vi "ResonanceAnalyzer.vi"() -> ()   [LabVIEW 2015]
uses:
  <vilib>/imath/engines/lvmath2/RunTimeEngine/Managers/WorkSpace/UID Generator.vi
  <vilib>/imath/engines/lvmath2/RunTimeEngine/RangeToken/NIMS_Range_R2 - Float.vi
  <instcachedir>/0/NIMS_Range_R2 - Float_98052C3F8D284261A146188355820AF0.lvgen/NIMS_Range_R2 - Float_98052C3F8D284261A146188355820AF0_000.vi
  <vilib>/imath/engines/lvmath2/RunTimeEngine/CommandStatement/MC_CommandStatement_break.vi
  <vilib>/imath/engines/lvmath2/RunTimeEngine/RunTimeType/NIMS_RunTimeType_From StrictType (excl LVString).vi
  <instcachedir>/0/NIMS_RunTimeType_From StrictType (excl LVString)_EB1C38A9BC5048DA9ABDA8F781E54D21.lvgen/NIMS_RunTimeType_From StrictType (excl LVString)_EB1C38A9BC5048DA9ABDA8F781E54D21_000.vi
  <vilib>/imath/engines/lvmath2/RunTimeEngine/LocalVariableDefStatement/MC_LocalVariableDefStatement_Display.vi
  <vilib>/imath/engines/lvmath2/RunTimeEngine/RowToken/NIMS_RowToken_M_SorRV.vi
  <instcachedir>/0/NIMS_RowToken_M_SorRV_0ECFFCDE6465458AAAF8A8ED2D6C8AF1.lvgen/NIMS_RowToken_M_SorRV_0ECFFCDE6465458AAAF8A8ED2D6C8AF1_003.vi
  <vilib>/imathl/engines/lvmath/Functions/Error Handling/Create Error.vi
  <instcachedir>/0/NIMS_RowToken_M_SorRV_0ECFFCDE6465458AAAF8A8ED2D6C8AF1.lvgen/NIMS_RowToken_M_SorRV_0ECFFCDE6465458AAAF8A8ED2D6C8AF1_002.vi
  <vilib>/imath/engines/lvmath2/RunTimeEngine/BuiltInFunctions/randnormal/NIMS_randnormal(1,I32).vi
  <vilib>/imath/engines/lvmath2/RunTimeEngine/ErrorHandling/NIMS_Error From Error Code.vi
  <vilib>/imath/engines/lvmath2/RunTimeEngine/NodeEndStatement/NIMS_NodeEndStatement_Get Vector.vi
  <instcachedir>/0/NIMS_NodeEndStatement_Get Vector_ED7FC4F6B50246F79D573C75B2E51AF8.lvgen/NIMS_NodeEndStatement_Get Vector_ED7FC4F6B50246F79D573C75B2E51AF8_003.vi
  <vilib>/imath/engines/lvmath2/RunTimeEngine/VariableToken/NIMS_VariableToken_CondDefined.vi
  <instcachedir>/0/NIMS_VariableToken_CondDefined_FE30D0A1BFB24F098D41DEBABFE96BE1.lvgen/NIMS_VariableToken_CondDefined_FE30D0A1BFB24F098D41DEBABFE96BE1_003.vi
  <instcachedir>/0/NIMS_NodeEndStatement_Get Vector_ED7FC4F6B50246F79D573C75B2E51AF8.lvgen/NIMS_NodeEndStatement_Get Vector_ED7FC4F6B50246F79D573C75B2E51AF8_001.vi
  <vilib>/imath/engines/lvmath/Functions/Error Handling/MergeErrorsWrapper.vi
  <vilib>/imath/engines/lvmath2/RunTimeEngine/Managers/SymbolTable/Clear UID.vi
  <vilib>/imath/engines/lvmath2/RunTimeEngine/NodeEndStatement/NIMS_NodeEndStatement_Output.vi
  <instcachedir>/0/NIMS_NodeEndStatement_Output_53EC0D466D134D7ABD903AC30B43404B.lvgen/NIMS_NodeEndStatement_Output_53EC0D466D134D7ABD903AC30B43404B_005.vi
  <vilib>/imath/engines/lvmath2/RunTimeEngine/ErrorHandling/NIMS_Finalize Error.vi
  <vilib>/Utility/file.llb/Read Delimited Spreadsheet (DBL).vi
  <vilib>/imath/engines/lvmath2/RunTimeEngine/Managers/SymbolTable/NIMS_WorkSpace.lvlib
panel:
  out "Results":T1={"Amplitude"=1.0125354246286684, "Q"=10.011231515184043, "Center Freq"=599.8902895404412}
  out "XY Graph":cluster{"freq":dbl[], "Array":dbl[]}[](graph)=[{"freq"=[400.0, 401.0, 402.0, 403.0, 404.0, 405.0, 406.0, 407.0, 408.0, 409.0, 410.0, 411.0, 412.0, 413.0, 414.0, 415.0, 416.0, 417.0, 418.0, 419.0, 420.0, 421.0, 422.0, 423.0, 424.0, 425.0, 426.0, 427.0, 428.0, 429.0, 430.0, 431.0, 432.0, 433.0, 434.0, 435.0, 436.0, 437.0, 438.0, 439.0, 440.0, 441.0, 442.0, 443.0, 444.0, 445.0, 446.0, 447.0, 448.0, 449.0, 450.0, 451.0, 452.0, 453.0, 454.0, 455.0, 456.0, 457.0, 458.0, 459.0, 460.0, 461.0, 462.0, 463.0, 464.0, 465.0, 466.0, 467.0, 468.0, 469.0, 470.0, 471.0, 472.0, 473.0, 474.0, 475.0, 476.0, 477.0, 478.0, 479.0, 480.0, 481.0, 482.0, 483.0, 484.0, 485.0, 486.0, 487.0, 488.0, 489.0, 490.0, 491.0, 492.0, 493.0, 494.0, 495.0, 496.0, 497.0, 498.0, 499.0, 500.0, 501.0, 502.0, 503.0, 504.0, 505.0, 506.0, 507.0, 508.0, 509.0, 510.0, 511.0, 512.0, 513.0, 514.0, 515.0, 516.0, 517.0, 518.0, 519.0, 520.0, 521.0, 522.0, 523.0, 524.0, 525.0, 526.0, 527.0, 528.0, 529.0, 530.0, 531.0, 532.0, 533.0, 534.0, 535.0, 536.0, 537.0, 538.0, 539.0, 540.0, 541.0, 542.0, 543.0, 544.0, 545.0, 546.0, 547.0, 548.0, 549.0, 550.0, 551.0, 552.0, 553.0, 554.0, 555.0, 556.0, 557.0, 558.0, 559.0, 560.0, 561.0, 562.0, 563.0, 564.0, 565.0, 566.0, 567.0, 568.0, 569.0, 570.0, 571.0, 572.0, 573.0, 574.0, 575.0, 576.0, 577.0, 578.0, 579.0, 580.0, 581.0, 582.0, 583.0, 584.0, 585.0, 586.0, 587.0, 588.0, 589.0, 590.0, 591.0, 592.0, 593.0, 594.0, 595.0, 596.0, 597.0, 598.0, 599.0, 600.0, 601.0, 602.0, 603.0, 604.0, 605.0, 606.0, 607.0, 608.0, 609.0, 610.0, 611.0, 612.0, 613.0, 614.0, 615.0, 616.0, 617.0, 618.0, 619.0, 620.0, 621.0, 622.0, 623.0, 624.0, 625.0, 626.0, 627.0, 628.0, 629.0, 630.0, 631.0, 632.0, 633.0, 634.0, 635.0, 636.0, 637.0, 638.0, 639.0, 640.0, 641.0, 642.0, 643.0, 644.0, 645.0, 646.0, 647.0, 648.0, 649.0, 650.0, 651.0, 652.0, 653.0, 654.0, 655.0, 656.0, 657.0, 658.0, 659.0, 660.0, 661.0, 662.0, 663.0, 664.0, 665.0, 666.0, 667.0, 668.0, 669.0, 670.0, 671.0, 672.0, 673.0, 674.0, 675.0, 676.0, 677.0, 678.0, 679.0, 680.0, 681.0, 682.0, 683.0, 684.0, 685.0, 686.0, 687.0, 688.0, 689.0, 690.0, 691.0, 692.0, 693.0, 694.0, 695.0, 696.0, 697.0, 698.0, 699.0, 700.0, 701.0, 702.0, 703.0, 704.0, 705.0, 706.0, 707.0, 708.0, 709.0, 710.0, 711.0, 712.0, 713.0, 714.0, 715.0, 716.0, 717.0, 718.0, 719.0, 720.0, 721.0, 722.0, 723.0, 724.0, 725.0, 726.0, 727.0, 728.0, 729.0, 730.0, 731.0, 732.0, 733.0, 734.0, 735.0, 736.0, 737.0, 738.0, 739.0, 740.0, 741.0, 742.0, 743.0, 744.0, 745.0, 746.0, 747.0, 748.0, 749.0, 750.0, 751.0, 752.0, 753.0, 754.0, 755.0, 756.0, 757.0, 758.0, 759.0, 760.0, 761.0, 762.0, 763.0, 764.0, 765.0, 766.0, 767.0, 768.0, 769.0, 770.0, 771.0, 772.0, 773.0, 774.0, 775.0, 776.0, 777.0, 778.0, 779.0, 780.0, 781.0, 782.0, 783.0, 784.0, 785.0, 786.0, 787.0, 788.0, 789.0, 790.0, 791.0, 792.0, 793.0, 794.0, 795.0, 796.0, 797.0, 798.0, 799.0, 800.0], "Array"=[0.10740244651787122, 0.15281838289829783, 0.08959115748735166, 0.14809526149818455, 0.13102686084532728, 0.1104993829827506, 0.1221783389006147, 0.15050889317348842, 0.12029736326487445, 0.13037718741363646, 0.15243658974820584, 0.1374153902648614, 0.10978943923875586, 0.11543254265874583, 0.116749384195053, 0.15255299393630767, 0.12857585311403671, 0.11097529559717934, 0.1350388671955145, 0.14129997658045362, 0.16703549012694668, 0.14056905939318204, 0.15670938293701409, 0.1745965004264096, 0.15263763075519182, 0.1538378456426476, 0.1655560882427844, 0.15042578416569982, 0.17077928893541036, 0.14546868063086157, 0.1284127118932754, 0.14499346079719164, 0.14922747914991136, 0.1776417666138386, 0.14486375149154065, 0.1514964505869006, 0.1423909822834546, 0.1221032080951852, 0.12573244654842436, 0.16394597483895484, 0.18819152291011748, 0.15653899730011506, 0.12231585004152735, 0.13837823070137883, 0.1820668469920245, 0.16117180400928585, 0.18404838769308257, 0.18388021368066343, 0.148855772839171, 0.16783333316882265, 0.15503774605936327, 0.16367980030790852, 0.1579857648450566, 0.18191502199890683, 0.18970595823297254, 0.1944117552163931, 0.17266173161962406, 0.1802135947011225, 0.17855434351423938, 0.20062811939961647, 0.20654642108343524, 0.2052027035839432, 0.14902958539641598, 0.1762033423674224, 0.18327011348703162, 0.2283954425279633, 0.21827276447564503, 0.17754461590565587, 0.1892535385196978, 0.17952124670585873, 0.20008031880994345, 0.18189891897781724, 0.19794893957248644, 0.17613003418044218, 0.2249405249742432, 0.2121694451348723, 0.236670289359744, 0.2122005230430719, 0.1991946566567743, 0.212989347219985, 0.1787092964007292, 0.23389290334086227, 0.21930355311221128, 0.2559430561689233, 0.2107510422017375, 0.2213373501904825, 0.23459650705845927, 0.23411604572589576, 0.24232120185154685, 0.2579793486248234, 0.2558574257254317, 0.20496503693873555, 0.23239561943384532, 0.20896666579796563, 0.2614634805616313, 0.2258417261954543, 0.2471379676293738, 0.29307296878981853, 0.26178804891270624, 0.28960879040736437, 0.2788051456775778, 0.2737419120741029, 0.2784378688053793, 0.27898009359666054, 0.2915181736906019, 0.3033190946663929, 0.3000947700143919, 0.29665578583792496, 0.27482781058991157, 0.276171909679604, 0.27867649313953385, 0.2900655139885531, 0.2847266539584309, 0.2827978296624287, 0.31246587606549975, 0.3182942076336981, 0.2996410250956576, 0.32466743458622577, 0.3200048633179981, 0.31396337632360016, 0.3383915715497288, 0.32037493481420787, 0.34373662643485814, 0.3766872010424195, 0.34832133013105215, 0.33889616380084375, 0.4074268521903415, 0.34953183194534726, 0.33611613987777045, 0.39974131071551966, 0.3566730066279571, 0.34703115551990643, 0.3968775547607246, 0.4043501402167882, 0.3761696888376735, 0.3948411944517424, 0.3690359877672123, 0.43399509946970144, 0.43673286069535106, 0.39641181561210903, 0.4137969831790379, 0.4617765348706966, 0.4726295604520662, 0.4261537242721796, 0.4514042366383567, 0.45426474364682407, 0.45154083243783616, 0.49668249205938647, 0.4672454873406263, 0.5048940014747391, 0.5130668244433702, 0.5416562561443161, 0.5268395198682813, 0.5320264594999139, 0.546074355673345, 0.5251244571563372, 0.5744842802378644, 0.581350604617343, 0.5795838749124972, 0.5623338651916296, 0.5935843524297746, 0.5894221188352807, 0.6062038075829269, 0.6417195251539344, 0.634690715231069, 0.651868808006857, 0.6677428951850922, 0.6633513933529221, 0.6926614547702747, 0.6789450971670071, 0.7004064565103679, 0.6988271486328266, 0.7249285790621133, 0.7576714767505519, 0.7933063177685261, 0.8042720699856534, 0.7740231288836648, 0.7908060031158608, 0.8348634973967137, 0.844537787339374, 0.8400940710471335, 0.8482714179186746, 0.8432113148306352, 0.8703815460446738, 0.8968823832449301, 0.8715528206370958, 0.9308369472650522, 0.946983134130226, 0.9331356861843558, 0.9310495156756244, 0.9578146226109034, 0.9899983028755162, 0.9934759739042415, 0.9865124430027351, 1.0198994221003552, 0.9793454680620476, 1.040723912454541, 1.0019829426536175, 0.9878851948437057, 0.9931436118790047, 0.9998997955421117, 1.0241340949804192, 0.9980604879191322, 1.0004059988811909, 0.9964311453849393, 1.035115606150817, 1.014821095046213, 0.9889263917806297, 1.0179292524113845, 0.9605549119859166, 0.9560504690148568, 0.922530600901802, 0.9022757533720215, 0.9183222779288016, 0.9048488262003115, 0.9071789367812199, 0.9289015802343044, 0.8485576784792067, 0.8417815720374748, 0.8631395677579252, 0.8802707620426905, 0.8239894591940262, 0.8194511336977124, 0.7907852548996013, 0.813393533100567, 0.7813841594826026, 0.7335140123481045, 0.7690250917543924, 0.7661270744942449, 0.7081428294002305, 0.7275011248548809, 0.7288470799197462, 0.7310329276991778, 0.6858348894016951, 0.6545573028680088, 0.6640132244545103, 0.644157127864353, 0.6291484828008138, 0.6394589009817717, 0.6067453989698446, 0.6532855868688, 0.6161204004806324, 0.6150443381543468, 0.604273501743808, 0.6142461968037111, 0.5478912448786132, 0.5436770383181866, 0.5595910875659509, 0.5663136233109691, 0.5726300741195651, 0.5374425496882539, 0.5331011268367872, 0.49814276248296235, 0.5168627643519728, 0.49766324611051416, 0.494509126918839, 0.44464226610264207, 0.46929064541696053, 0.5205436518966415, 0.47456930528748426, 0.4273781407761661, 0.500119758518092, 0.5073860051476381, 0.4522174778467483, 0.43540532391181086, 0.4277470264905283, 0.45017848944633887, 0.38725813822260935, 0.43674588843293044, 0.42458002025502534, 0.4127836504534946, 0.4103666012150693, 0.40156767957870654, 0.39257867428810883, 0.40667705195073284, 0.43063546042850814, 0.3659919078706112, 0.40972523395198057, 0.40736834646343606, 0.4007217107777696, 0.3775120158678112, 0.35347247408739463, 0.3665994653344173, 0.35075199676799695, 0.32756109923258453, 0.37819715452738345, 0.35086941336678446, 0.35364004526844284, 0.3508398401104885, 0.3278260030576613, 0.32606974975065, 0.36441220206503216, 0.3440542864177623, 0.33103347985615655, 0.34576209714919515, 0.29092039816816706, 0.322274373671659, 0.3289061621350945, 0.30706296086408164, 0.3356218820756341, 0.32657661683896744, 0.2718225279989093, 0.32117955239798424, 0.30421160254751883, 0.27488395739312743, 0.2699908334822933, 0.2974915668952296, 0.28030899970393053, 0.27808804851581603, 0.24958907402046104, 0.27752879200285546, 0.28798032098818105, 0.2899865558922329, 0.254155342047928, 0.27433746535894193, 0.2966394614788142, 0.2650608715264895, 0.25932977780652283, 0.26487880078924225, 0.28141762463064746, 0.24233375708797547, 0.26702591219274524, 0.27655649784368713, 0.2749902813664165, 0.30379696818985197, 0.23350986845042287, 0.2914434978036537, 0.2548922376708591, 0.23154428185303677, 0.2693647169174003, 0.246150843221038, 0.24582181840925713, 0.2683660789256584, 0.25505675230040076, 0.25502826942985396, 0.27409213618113265, 0.22923011909348115, 0.23902506489589356, 0.2263346242039908, 0.21302480728051618, 0.23727434998850835, 0.2262192765545401, 0.21310004964379087, 0.248655475562663, 0.20180136113191977, 0.2122401027267436, 0.2509455407040858, 0.230264588483497, 0.20250360523920458, 0.22731653665623414, 0.2490361788808062, 0.22643826343509388, 0.22968142184378812, 0.228650289735457, 0.17747612924159473, 0.19587939404704874, 0.2365709003275931, 0.2207676659030181, 0.22120487822560841, 0.18393665061567777, 0.21599364522205494, 0.19373202283935284, 0.23389465084970545, 0.22983528539400916, 0.19334916599901192, 0.19245765890172797, 0.22578301105299753, 0.19775413579077106, 0.17816726939045804, 0.18966882935080356, 0.18760245648961316, 0.1914780125451503, 0.23305415087844095, 0.2143436771140928, 0.18712407047353985, 0.18032134679831235, 0.19347382576694527, 0.21362119150828224, 0.20185364505963843, 0.20433145754719834, 0.20329667400716067, 0.19029914718681923, 0.1591216111307436, 0.19208811147022664, 0.1926714623146115, 0.1597415120392497, 0.1852098930696274, 0.18637084164384937, 0.19146388692811167, 0.20547364695786818, 0.17863226190779827, 0.15695795749571714, 0.18214109732385403, 0.17367128443407268, 0.1613401334142838, 0.1700049889142177, 0.17999562799846414, 0.18759946320178397, 0.19154195290156165, 0.17609562635859496, 0.16345341866704946]}, ...(2 in all)]
  in  "Tab Control":enum32{"Simulated", "Experiment"}(tab)
  in  "df":dbl=0.314159
  in  "Q":dbl=10.0
  in  "Center Freq":dbl=600.0
  in  "Start Freq":dbl=400.0
  in  "End Freq":dbl=800.0
  in  "Noise Level":dbl=0.02
  in  "Filename":path
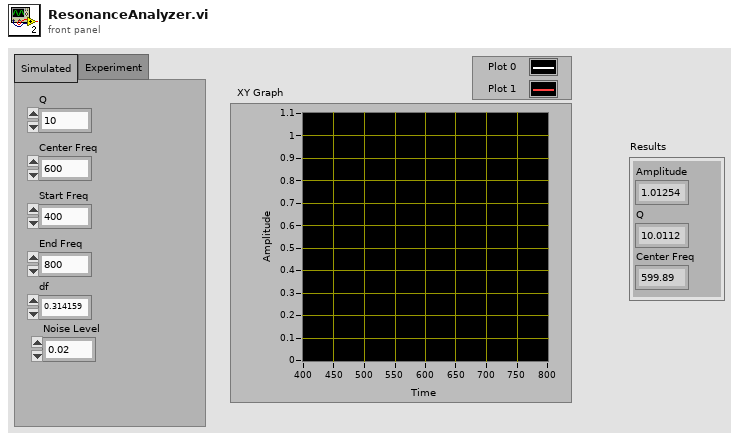
[diagram p1: front panel]
types:
  T1 = cluster{"Amplitude":dbl, "Q":dbl, "Center Freq":dbl}
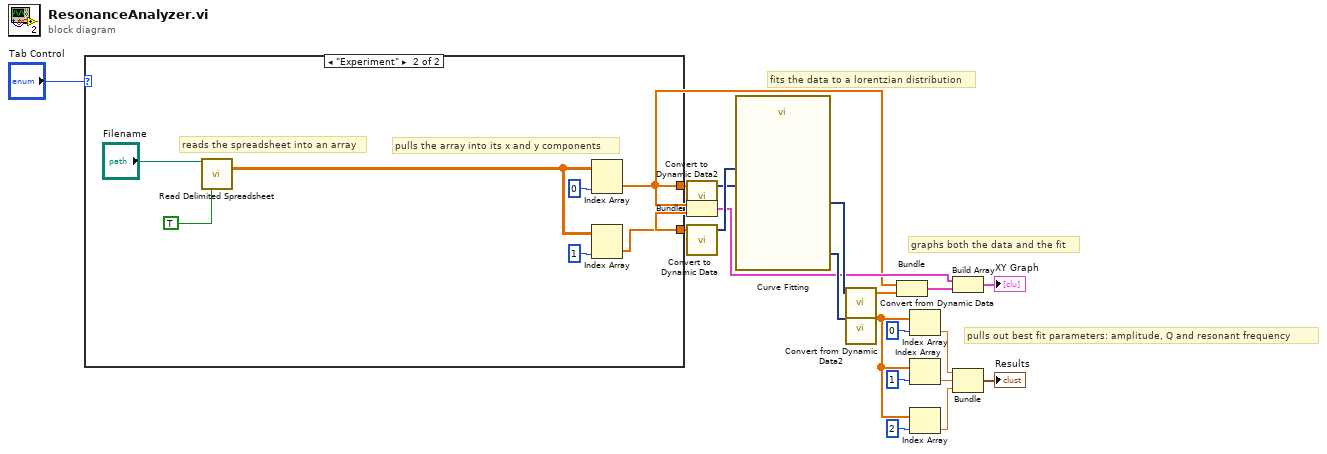
[diagram p0: block diagram]
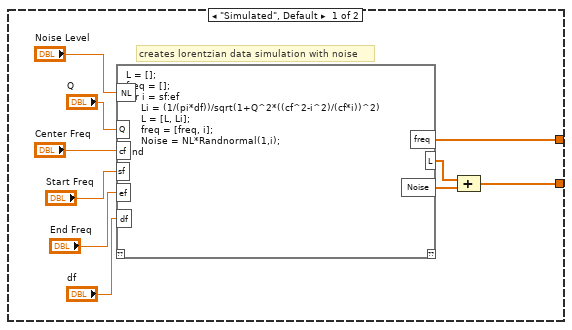
[diagram p2: hidden frame]
diagram:
  # "graphs both the data and the fit"
  # "pulls out best fit parameters: amplitude, Q and resonant frequency"
  # "fits the data to a lorentzian distribution"
  n1 = case shown="\"Experiment\"" "Tab Control" {
    tunnel: [w21 w253] -> w1
    tunnel: [w20 w256] -> w2
    frame "Simulated", Default {
      # "creates lorentzian data simulation with noise"
      n2 = mathscript code="L = [];\nfreq = [];\nfor i = sf:ef \n     Li = (1/(pi*df))/sqrt(1+Q^2*((cf^2-i^2)/(cf*i))^2)\n     L = [L, Li];\n     freq = [freq, i];\n     Noise = NL*Randnormal(1,i);\nend"("cf"="Center Freq", "Q"="Q", "sf"="Start Freq", "ef"="End Freq", "NL"="Noise Level", "df"="df") -> ("freq"=w20:dbl[], "L"=w23:dbl[], "Noise"=w24:dbl[])  [unwired: 1 in, 1 out]
      n3 = Compound Arithmetic op=ADD(w23, w24) -> (w21:dbl[])
    }
    frame "Experiment" {
      # "pulls the array into its x and y components"
      # "reads the spreadsheet into an array"
      n4 = call-poly <vilib>:"Read Delimited Spreadsheet.vi"("file path (dialog if empty)"="Filename", "transpose? (F)"=TRUE) -> ("all rows"=w257:dbl[][])  [unwired: 8 in, 5 out]
      n5 = Index Array(array=w257, index (col)=0 ("index (row)")) -> (element=w256:dbl[])  [unwired: 1 in]
      n6 = Index Array(array=w257, index (col)=1 ("index (row)")) -> (element=w253:dbl[])  [unwired: 1 in]
    }
  }
  n7 = call "Convert to Dynamic Data2"("Array"=w2) -> ("Dynamic Data Type"=w17:dynamicdata)  [unwired: 3 in]
  n8 = Bundle("all rows"=w2, "all rows"=w1) -> (w3:cluster{"all rows":dbl[], "all rows":dbl[]})  [unwired: 1 in]
  n9 = call "Convert to Dynamic Data"("Array"=w1) -> ("Dynamic Data Type"=w18:dynamicdata)  [unwired: 3 in]
  n10 = call "Curve Fitting"("Locations"=w17, "Signals"=w18) -> ("best fit"=w15:dynamicdata, "non-linear coefficients"=w12:dynamicdata)  [unwired: 5 in, 3 out]
  n11 = call "Convert from Dynamic Data"("Dynamic Data Type"=w15) -> ("Array"=w14:dbl[])  [unwired: 3 in]
  n12 = call "Convert from Dynamic Data2"("Dynamic Data Type"=w12) -> ("Array"=w11:dbl[])  [unwired: 3 in]
  n13 = Bundle("all rows"=w2, "Array"=w14) -> (w16:cluster{"all rows":dbl[], "Array":dbl[]})  [unwired: 1 in]
  n14 = Index Array(array=w11, index=0) -> (element=w7:dbl)
  n15 = Index Array(array=w11, index=1) -> (element=w6:dbl)
  n16 = Index Array(array=w11, index=2) -> (element=w5:dbl)
  n17 = Build Array(w3, w16) -> (→"XY Graph":cluster{"all rows":dbl[], "Array":dbl[]}[])
  n18 = Bundle(w7, w6, w5) -> (→"Results":cluster{dbl, dbl, dbl})  [unwired: 1 in]
